vi "Counter_to_Boolean.vi"(5 "Counter":u32, 11 "Error In":errorcluster) -> (6 "ON/OFF":bool, 15 "Error Out":errorcluster)   [LabVIEW 2016]
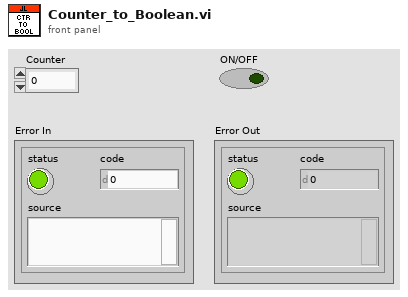
[diagram p1: front panel]
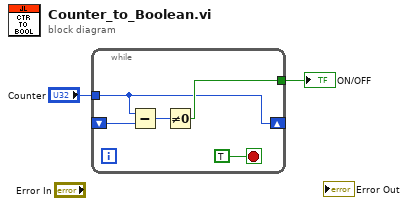
[diagram p0: block diagram]
diagram:
  n1 = while {
    tunnel: "Counter" -> [w4]
    shift-right: [w4] -> _
    shift-left: _ -> [w3]
    tunnel: [w5] -> w1
    stop <- TRUE stop-if-true
    n2 = Subtract(x=w4, y=w3) -> (x-y=w6:u32)
    n3 = Not Equal To 0?(x=w6) -> (x != 0?=w5:bool)
  }
  "ON/OFF" <- w1
